vi "Discover and Search Temp.vi"() -> ()   [LabVIEW 2014]
uses:
  <vilib>/rvi/Emulation/niFpgaGetClockAttributes.vi
  <vilib>/rvi/Emulation/niFpgaSctlEmulationGetInTimedLoop.vi
  <vilib>/rvi/Emulation/niFpgaEmulationReportErrorSimple.vi
  <vilib>/rvi/Emulation/niFpgaCriticalErrorInLSC.vi
  <vilib>/rvi/eio/common/nirviEmuTemplateMethod_errors.vi
  <vilib>/eio/EIONode/EIONode.xnode
  Sub VIs/Maxim 1-Wire/Maxim 1-Wire.lvlib
panel:
  in  "RelayIO":bool
  out "Numeric":i32
  out "Temperature Array":u16[](array[numeric]) format="%x"
  out "Error Out":errorcluster
  out "ROM Array":u64[](array[numeric]) format="%x"
  in  "Error In":errorcluster
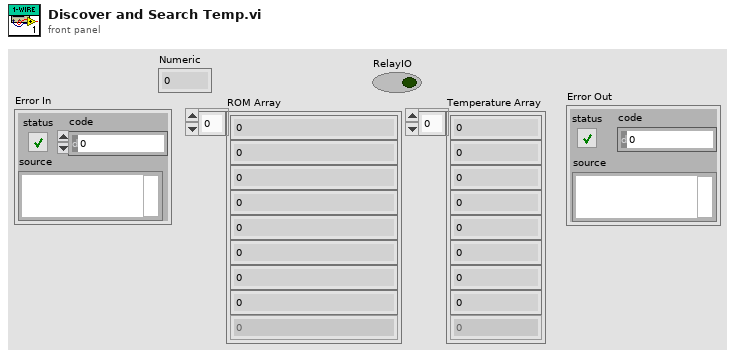
[diagram p1: front panel]
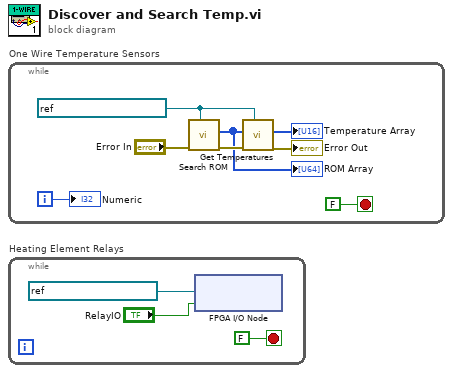
[diagram p0: block diagram]
diagram:
  n1 = while "One Wire Temperature Sensors" {
    i -> [w3]
    stop <- FALSE stop-if-true
    w2 = refnum<k21> "ConnectorA/DIO15" ("1-Wire DIO Pin")
    n2 = call "Search ROM.vi"("1-Wire DIO Pin"=w2, "Error In"="Error In") -> ("Error Out"=w5:errorcluster, "ROM Array"=w4:u64[])  [unwired: 7 in, 1 out]
    "ROM Array" <- w4
    n3 = call "Get Temperatures.vi"("1-Wire DIO Pin"=w2, "error in (no error)"=w5, "ROM Array"=w4) -> ("error out"=→"Error Out":errorcluster, "Temperature Array"=→"Temperature Array":u16[])  [unwired: 7 in]
    "Numeric" <- w3
  }
  n4 = while "Heating Element Relays" {
    stop <- FALSE stop-if-true
    n5 = xnode "FPGA I/O Node"("I/O Item"="RelayIO", "FPGA I/O In"=refnum<k21> "ConnectorA/DIO14" ("1-Wire DIO Pin")) -> ()  [unwired: 1 out]
  }
